vi "demo.vi"() -> ()   [LabVIEW 2018]
uses:
  sheep/Sheep.lvclass
  tiger/Tiger.lvclass
  animal/Animal.lvclass
panel:
  out "Array":string[](array[string])
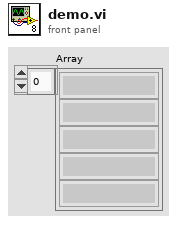
[diagram p1: front panel]
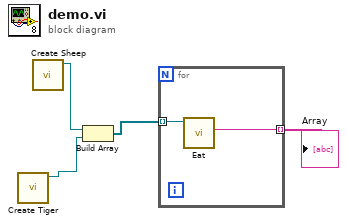
[diagram p0: block diagram]
diagram:
  n1 = call "Create Tiger.vi"() -> ("output cluster"=w3:refnum<class "Tiger.lvclass">)  [unwired: 11 in]
  n2 = call "Create Sheep.vi"() -> ("Sheep.lvclass"=w4:refnum<class "Sheep.lvclass">)  [unwired: 11 in]
  n3 = Build Array(w4, w3) -> (w2:refnum<class "Animal.lvclass">[])
  n4 = for {
    tunnel: w2 -> [w6] mode=indexing
    tunnel: [w5] -> w1 mode=indexing
    n5 = call-dynamic "Eat.vi"("Animal in"=w6) -> ("String 2"=w5:string)  [unwired: 8 in, 2 out]
  }
  "Array" <- w1
